vi "Classes_Get All.vi"(8 "error in":errorcluster) -> (0 "error out":errorcluster, 3 "All Classes Tree Sorted":T1(array[cluster]))   [LabVIEW 2023]
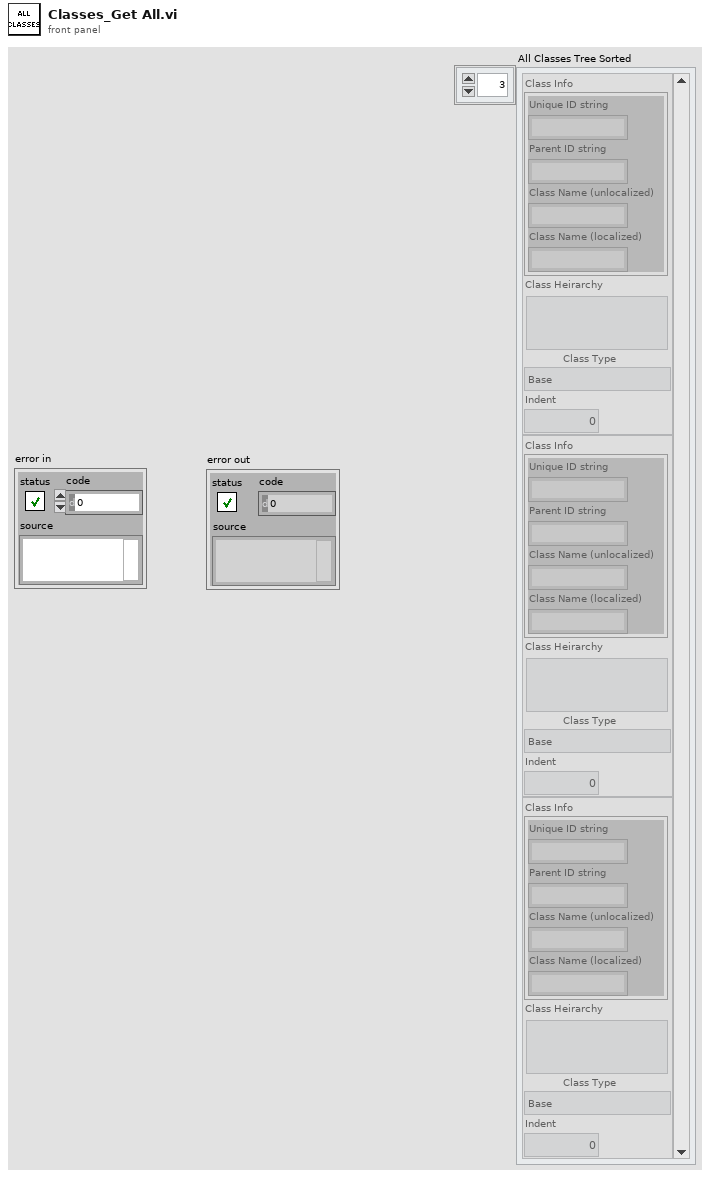
[diagram p1: front panel]
types:
  T1 = cluster{"Class Info":cluster{"Unique ID string":string, "Parent ID string":string, "Class Name (unlocalized)":string, "Class Name (localized)":string}, "Class Heirarchy":string, "Class Type":enum16{"Unknown", "Base", "Scripting", "Private", "Deprecated", "None", "Divider"}, "Indent":u32}[]
  T2 = cluster{"Unique ID string":string, "Parent ID string":string, "Class Name (unlocalized)":string, "Class Name (localized)":string}[]
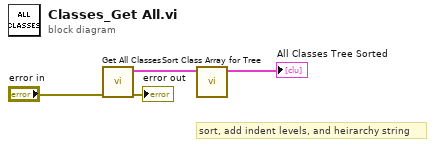
[diagram p0: block diagram]
diagram:
  # "sort, add indent levels, and heirarchy string"
  n1 = call "Get All Classes.vi"("error in (no error)"="error in") -> ("error out"=→"error out":errorcluster, "VI Server Classes[]"=w3:T2)  [unwired: 9 in]
  n2 = call "Sort Class Array for Tree.vi"("All Classes"=w3) -> ("All Classes Tree Sorted"=→"All Classes Tree Sorted":T1)  [unwired: 10 in]
